vi "Action - XNET CAN Reader.vi"(7 "PackageID":i32, 8 "error in":errorcluster, 11 "CAN Configuration":T1={"CAN Interface"="CAN1", "XNET Cluster"="ManyXnetChannels", "#Signals"=0, "Sample Rate (Hz)"=100.0} {"Sample Rate (Hz)" format="%#_13g"}) -> (0 "error out":errorcluster)   [LabVIEW 2021, in "XNET-CAN-Signal-Logger.lvlib"]
uses:
  XNET-CAN-Signal-Logger.lvlib
  Typedef/Def-CAN Port Configuration.ctl
  Typedef/Def-Data Queue Type.ctl
  Global Variables.vi
  <vilib>/xnet/xnet.llb/XNET Create Session (Signal Input Waveform).vi
  <vilib>/xnet/xnet.llb/XNET Read (Signal Waveform) .vi
  <resource>/objmgr/xnet.rc
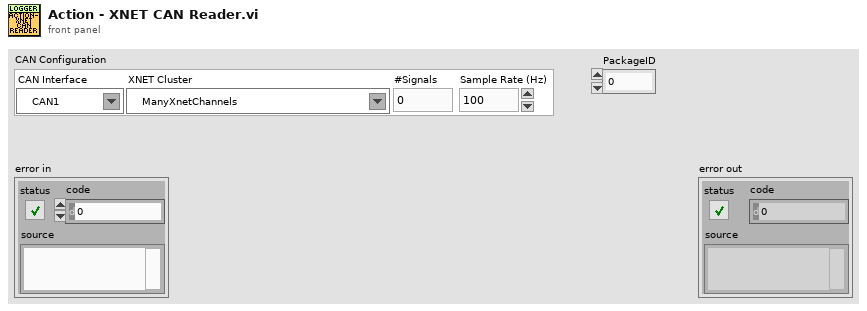
[diagram p1: front panel]
types:
  T1 = typedef "XNET-CAN-Signal-Logger.lvlib/Def-CAN Port Configuration.ctl" = cluster{"CAN Interface":refnum<k21>, "XNET Cluster":refnum<k21>, "#Signals":i32, "Sample Rate (Hz)":dbl}
  T2 = typedef "XNET-CAN-Signal-Logger.lvlib/Def-Data Queue Type.ctl" = cluster{"PackageID":i32, "Data":waveform(dbl)[]}
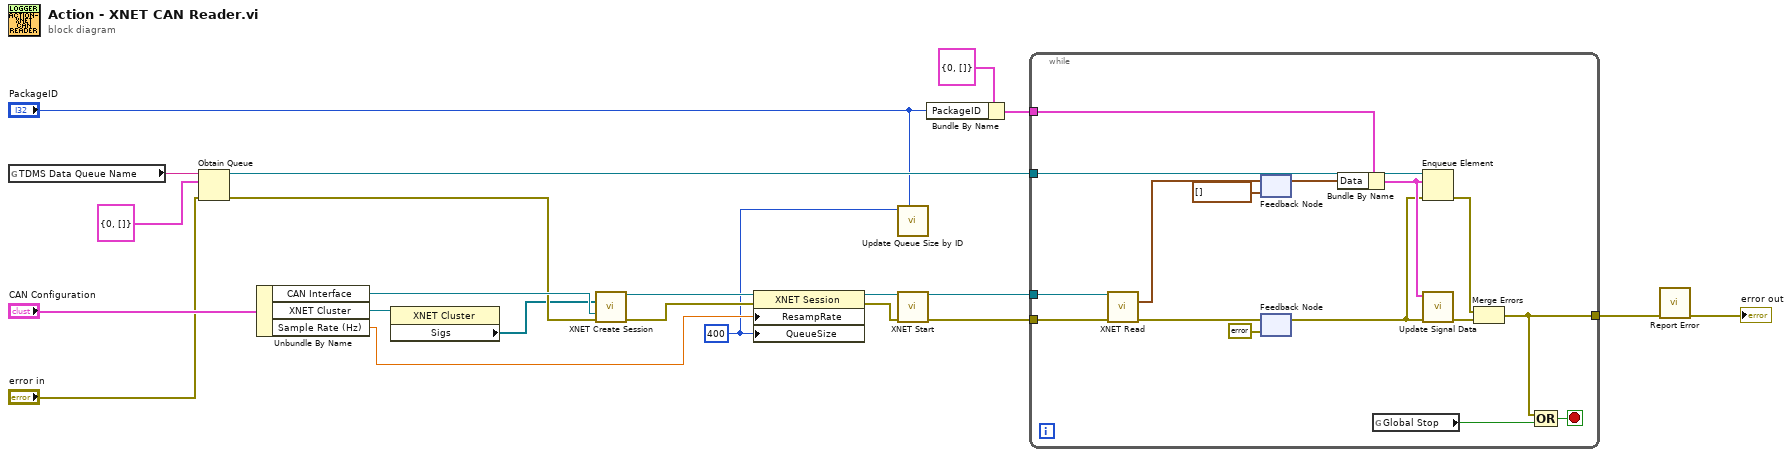
[diagram p0: block diagram]
diagram:
  w1 = u32 400 ("Queue Size")
  n1 = global read "Global Variables.vi" "TDMS Data Queue Name"() -> (w11:string)
  n2 = Obtain Queue(name (unnamed)=w11, element data type=T2 {"PackageID"=0, "Data"=[]} ("Data Queue Type"), error in (no error)="error in") -> (queue out=w9:refnum<queue>, error out=w7:errorcluster)  [unwired: 2 in, 1 out]
  n3 = Unbundle By Name("CAN Configuration") -> ("CAN Interface"=w16:refnum<k21>, "XNET Cluster"=w17:refnum<k21>, "Sample Rate (Hz)"=w2:dbl)
  n4 = property class="XNET Cluster"(reference=w17) -> ("Sigs"=w3:refnum<k21>[])  [unwired: 1 in, 2 out]
  n5 = call-poly <vilib>:"XNET Create Session.vi"("signal list"=w3, "interface"=w16, "error in (no error)"=w7) -> ("session out"=w22:refnum<k21>, "error out"=w21:errorcluster)  [unwired: 11 in]
  n6 = property class="XNET Session"(reference=w22, error in=w21, "ResampRate"=w2, "QueueSize"=w1) -> (reference out=w20:refnum<k21>, error out=w19:errorcluster)
  n7 = call "Update Queue Size by ID.vi"("PackageID"="PackageID", "Queue Size"=w1) -> ()  [unwired: 9 in, 1 out]
  n8 = call <vilib>:"XNET Start.vi"("session in"=w20, "error in (no error)"=w19) -> ("session out"=w15:refnum<k21>, "error out"=w14:errorcluster)  [unwired: 12 in]
  n9 = Bundle By Name(cluster=T2 {"PackageID"=0, "Data"=[]} ("element"), "PackageID"="PackageID") -> (w12:T2)
  n10 = while {
    tunnel: w9 -> [w36]
    tunnel: w15 -> [w37]
    tunnel: w14 -> [w33]
    tunnel: w12 -> [w35]
    tunnel: [w27] -> w5
    stop <- w34 stop-if-true
    n11 = call-poly <vilib>:"XNET Read.vi"("session in"=w37, "error in (no error)"=w33) -> ("data"=w32:waveform(dbl)[], "error out"=w30:errorcluster)  [unwired: 11 in, 1 out]
    n12 = feedback-in #1(w32) -> ()
    n13 = feedback #1(waveform(dbl)[] [] ("data")) -> (w26:waveform(dbl)[])
    n14 = feedback-in #2(w30) -> ()
    n15 = feedback #2(errorcluster {"status"=FALSE, "code"=0, "source"=""} ("error out")) -> (w25:errorcluster)
    n16 = Bundle By Name(cluster=w35, "Data"=w26) -> (w31:T2)
    n17 = global read "Global Variables.vi" "Global Stop"() -> (w38:bool)
    n18 = Enqueue Element(queue=w36, element=w31, error in (no error)=w25) -> (error out=w28:errorcluster)  [unwired: 1 in, 2 out]
    n19 = call "Update Signal Data.vi"("error in"=w25, "Data"=w31) -> ("error out"=w29:errorcluster)  [unwired: 9 in]
    n20 = Merge Errors(w28, w29) -> (w27:errorcluster)
    n21 = Compound Arithmetic op=OR(w27, w38) -> (w34:bool)
  }
  n22 = call "Report Error.vi"("error in (no error)"=w5) -> ("error out"=→"error out":errorcluster)  [unwired: 10 in]
